vi "2.vi"(0 "x1":dbl, 5 "x2":dbl, 7 "y1":dbl, 9 "y2":dbl, 11 "error in (no error)":errorcluster) -> (4 "d":dbl, 15 "error out":errorcluster)   [LabVIEW 2020]
panel:
  # "d=v(x1 – x2)² + (y1 – y2)²"
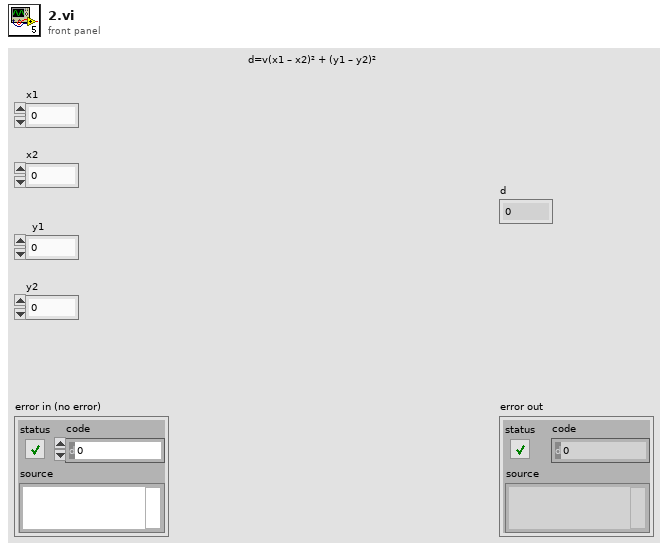
[diagram p1: front panel]
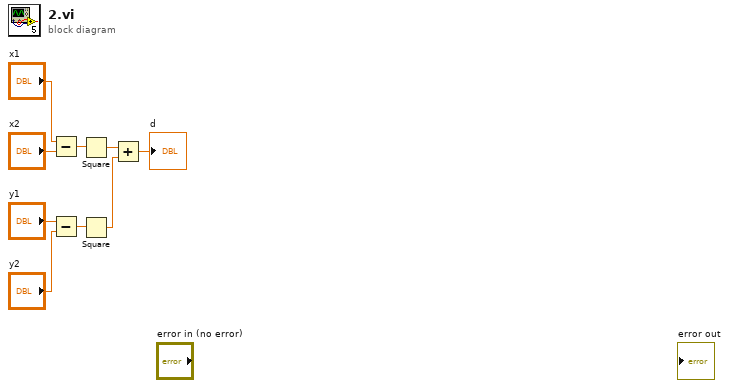
[diagram p0: block diagram]
diagram:
  n1 = Subtract(x="x1", y="x2") -> (x-y=w5:dbl)
  n2 = Subtract(x="y1", y="y2") -> (x-y=w4:dbl)
  n3 = Square(x=w5) -> (x^2=w3:dbl)
  n4 = Square(x=w4) -> (x^2=w2:dbl)
  n5 = Add(x=w3, y=w2) -> (x+y=→"d":dbl)
